vi "Write T start stop.vi"(8 "error in (no error)":errorcluster, 11 "Heater in":refnum<class "Heater_v2.lvclass">) -> (0 "error out":errorcluster, 3 "Heater out":refnum<class "Heater_v2.lvclass">)   [LabVIEW 2019, in "Heater_v2.lvclass"]
uses:
  Heater_v2.lvclass
  C:/my_projects/projects/Algorithms/Labview/19/Heating/heating1/ZM_state/HE_ZM_state.lvclass
  Heater_v2.lvclass/Heater_v2.ctl
  REG/HE_reg.lvclass/HE_reg.ctl
  Reg/PID/PID SP Limiter/PID SP Limiter.lvclass/PID SP Limiter.ctl
  ZM_state/HE_ZM_state.lvclass/HE_ZM_state.ctl
  Reg/PID/PID SP Limiter/PID SP Limiter.lvclass
  ZM_state/HE_ZM_state.lvclass
  REG/HE_reg.lvclass
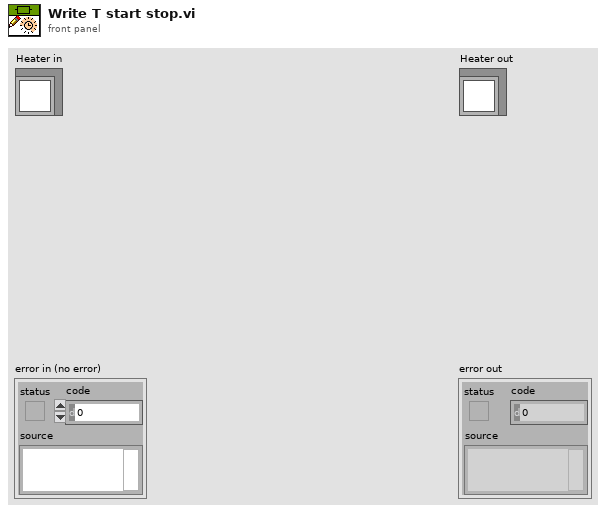
[diagram p1: front panel]
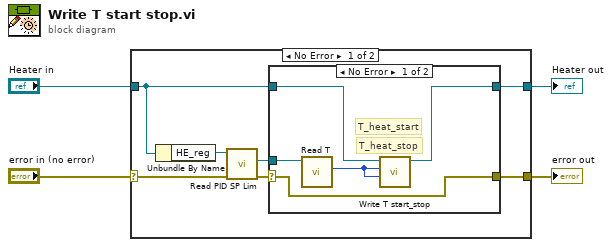
[diagram p0: block diagram]
diagram:
  n1 = case shown="No Error" "error in (no error)" {
    selector: "error in (no error)" -> [w7 w20]
    tunnel: [w9 w20] -> w3
    tunnel: [w10 w19] -> w1
    tunnel: "Heater in" -> [w11 w19]
    frame No Error {
      n2 = Unbundle By Name(w11) -> ("HE_reg"=w8:refnum<class "HE_reg.lvclass">)
      n3 = call "Read PID SP Lim.vi"("error in (no error)"=w7, "HE_reg in"=w8) -> ("error out"=w6:errorcluster, "PID SP Limiter"=w5:refnum<class "PID SP Limiter.lvclass">)  [unwired: 7 in, 1 out]
      n4 = case shown="No Error" w6 {
        selector: w6 -> [w12 w17]
        tunnel: w5 -> [w16 _]
        tunnel: w11 -> [w14 w18]
        tunnel: [w13 w18] -> w10
        tunnel: [w12 w17] -> w9
        frame No Error {
          # "T_heat_stop"
          # "T_heat_start"
          n5 = call "Read T.vi"("PID SP Limiter in"=w16) -> ("T"=w15:u32)  [unwired: 9 in, 1 out]
          n6 = call "Write T start_stop.vi"("T_heat_stop"=w15, "T_heat_start"=w15, "HE_ZM_state in"=w14) -> ("HE_ZM_state out"=w13:refnum<class "Heater_v2.lvclass">)  [unwired: 8 in]
        }
        frame Error {
        }
      }
    }
    frame Error {
    }
  }
  "error out" <- w3
  "Heater out" <- w1
